vi "Stop Command.vi"(8 "error in (no error)":errorcluster, 10 "Is Command Finished?":bool, 11 "System Actor in":refnum<class "System Actor.lvclass">) -> (0 "error out":errorcluster, 3 "System Actor out":refnum<class "System Actor.lvclass">)   [LabVIEW 2014, in "Robot Actor Framework.lvlib" / "System Actor.lvlib" / "System Actor.lvclass"]
uses:
  System Actor.lvclass
  <vilib>/ActorFramework/Message Enqueuer/Message Enqueuer.lvclass
  System Actor.lvclass/System Actor.ctl
  <vilib>/ActorFramework/Stop Msg/Stop Msg.lvclass/Stop Msg.ctl
  <vilib>/ActorFramework/Message Enqueuer/Message Enqueuer.lvclass/Message Enqueuer.ctl
  <vilib>/ActorFramework/Message Enqueuer/Enqueue Critical.vi
  <vilib>/ActorFramework/Message Priority Queue/Priority Enqueue.vi
  <vilib>/ActorFramework/Stop Msg/Stop Msg.lvclass
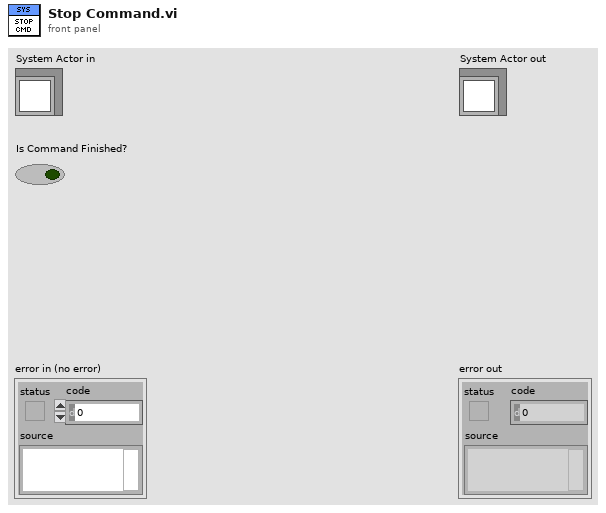
[diagram p1: front panel]
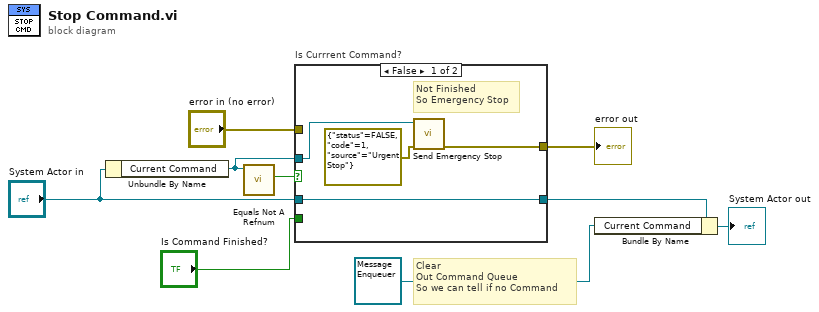
[diagram p0: block diagram]
diagram:
  # "Clear\nOut Command Queue\nSo we can tell if no Command"
  n1 = Unbundle By Name("System Actor in") -> ("Current Command"=w5:refnum<class "Message Enqueuer.lvclass">)
  n2 = call <vilib>:"Equals Not A Refnum.vi"("Message Enqueuer"=w5) -> ("Not a refnum?"=w4:bool)  [unwired: 10 in]
  n3 = case "Is Currrent Command?" shown="False" w4 {
    tunnel: w5 -> [w13 _]
    tunnel: [w12 w15] -> w3
    tunnel: "Is Command Finished?" -> [_ _]
    tunnel: "System Actor in" -> [w12 w15]
    tunnel: [w10 w14] -> w2
    tunnel: "error in (no error)" -> [_ w14]
    frame False {
      # "Not Finished\nSo Emergency Stop"
      n4 = call <vilib>:"Send Emergency Stop.vi"("error in (no error)"=errorcluster {"status"=FALSE, "code"=1, "source"="Urgent Stop"}, "Message Enqueuer"=w13) -> ("error out"=w10:errorcluster)  [unwired: 9 in]
    }
    frame True {
      # "Command Queue Is\nNot Valid so No Command\nTo Stop"
    }
  }
  "error out" <- w2
  n5 = Bundle By Name(cluster=w3, "Current Command"=refnum<class "Message Enqueuer.lvclass"> refnum ("Command Queue")) -> (→"System Actor out":refnum<class "System Actor.lvclass">)
